vi "MOPX2 Engine.vi"(8 "Operation Selection":T1, 9 "Main Parent  MO4J":u16[][](array[numeric]), 10 "Secondary Parent Schedule":u16[](array[numeric]), 11 "Main Parent Schedule":u16[](array[numeric])) -> (3 "Child Schedule":u16[](array[numeric]))   [LabVIEW 2013, in "GA.lvclass"]
uses:
  GA.lvclass
  Controls/MPOX2 Operation Selection Rule.ctl
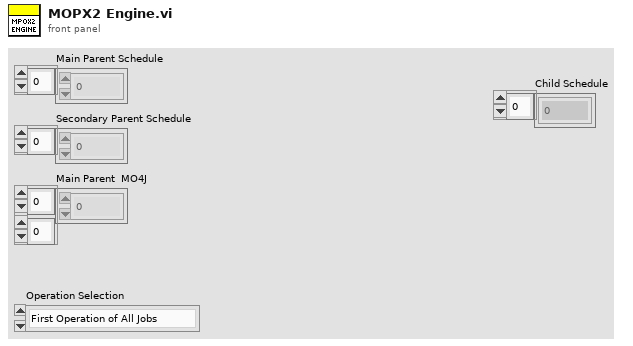
[diagram p1: front panel]
types:
  T1 = typedef "GA.lvclass/MPOX2 Operation Selection Rule.ctl" = enum16{"First Operation of All Jobs", "Random"}
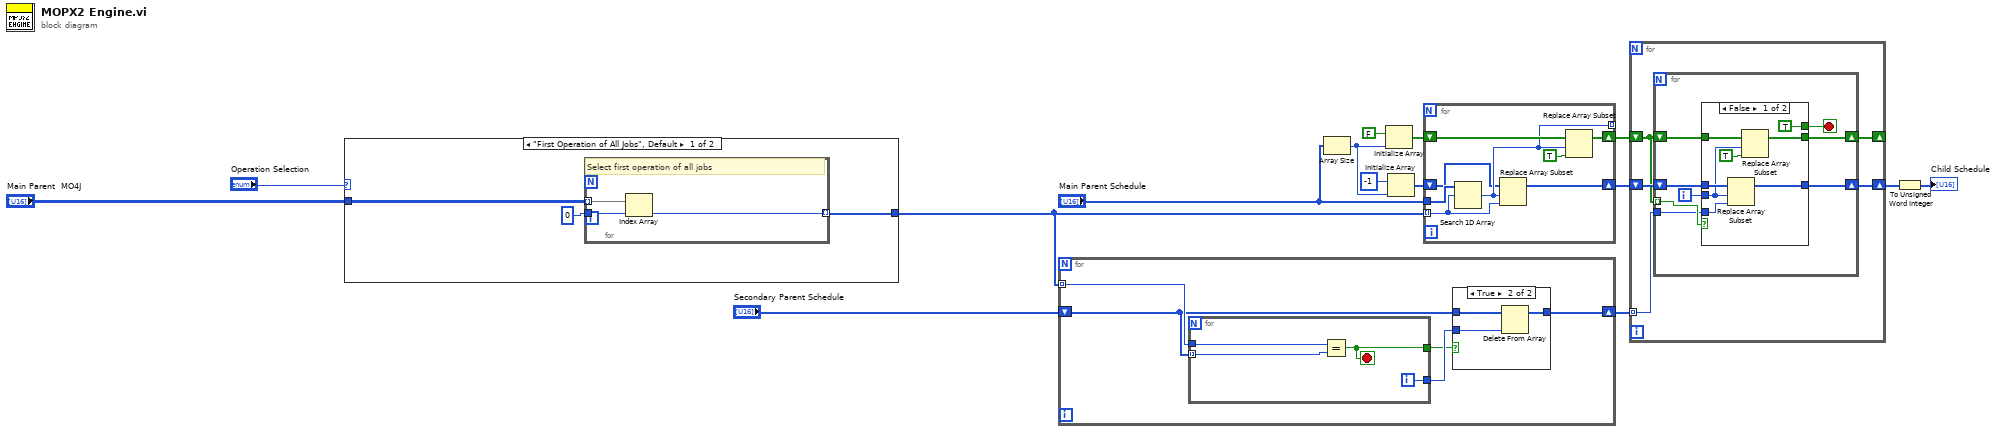
[diagram p0: block diagram]
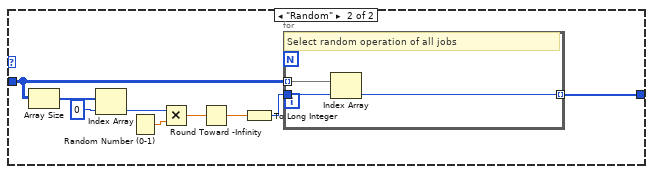
[diagram p2: hidden frame]
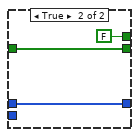
[diagram p3: hidden frame]
diagram:
  n1 = case shown="\"First Operation of All Jobs\", Default" "Operation Selection" {
    tunnel: "Main Parent  MO4J" -> [w18 w30]
    tunnel: [w17 w22] -> w2
    frame "First Operation of All Jobs", Default {
      n2 = for {
        tunnel: w18 -> [w21] mode=indexing
        tunnel: [w20] -> w17 mode=indexing
        tunnel: 0 ("index") -> [w19]
        # "Select first operation of all jobs"
        n3 = Index Array(array=w21, index=w19) -> (element=w20:u16)
      }
    }
    frame "Random" {
      n4 = Array Size(array=w30) -> (size(s)=w29:i32[])
      n5 = Index Array(array=w29, index=0) -> (element=w27:i32)
      n6 = Random Number (0-1)() -> (number: 0 to 1=w26:dbl)
      n7 = Multiply(x=w27, y=w26) -> (x*y=w25:dbl)
      n8 = Round Toward -Infinity(1:w25) -> (0:w24:dbl)
      n9 = To Long Integer(number=w24) -> (32bit integer=w23:i32)
      n10 = for {
        tunnel: w30 -> [w33] mode=indexing
        tunnel: [w32] -> w22 mode=indexing
        tunnel: w23 -> [w31]
        # "Select random operation of all jobs"
        n11 = Index Array(array=w33, index=w31) -> (element=w32:u16)
      }
    }
  }
  n12 = for {
    tunnel: w2 -> [w38] mode=indexing
    shift-right: [w35] -> w5
    shift-left: "Secondary Parent Schedule" -> [w37]
    n13 = for {
      tunnel: w37 -> [w45] mode=indexing
      tunnel: w38 -> [w46]
      tunnel: [w44] -> w36
      tunnel: [w43] -> w34
      i -> [w44]
      stop <- w43 stop-if-true
      n14 = Equal?(x=w46, y=w45) -> (x = y?=w43:bool)
    }
    n15 = case shown="True" w34 {
      tunnel: w37 -> [w39 w42]
      tunnel: w36 -> [_ w41]
      tunnel: [w39 w40] -> w35
      frame False {
      }
      frame True {
        n16 = Delete From Array(array=w42, index=w41) -> (array with subset deleted=w40:u16[])  [unwired: 1 in, 1 out]
      }
    }
  }
  n17 = Array Size(array="Main Parent Schedule") -> (size(s)=w11:i32)
  n18 = Initialize Array(FALSE, w11) -> (w13:bool[])
  n19 = Initialize Array(-1, w11) -> (w9:i32[])
  n20 = for {
    tunnel: "Main Parent Schedule" -> [w54]
    tunnel: w2 -> [w50] mode=indexing
    tunnel: [w51] -> _ mode=indexing
    shift-right: [w47] -> w7
    shift-left: w13 -> [w53]
    shift-right: [w48] -> w6
    shift-left: w9 -> [w49]
    n21 = Search 1D Array(1D array=w54, element=w50) -> (index of element=w51:i32)  [unwired: 1 in]
    n22 = Replace Array Subset(array=w49, new element=w50, index=w51) -> (w48:i32[])
    n23 = Replace Array Subset(array=w53, new element=TRUE ("new element/subarray"), index=w51) -> (w47:bool[])
  }
  n24 = for {
    tunnel: w5 -> [w59] mode=indexing
    shift-right: [w57] -> w4
    shift-left: w6 -> [w58]
    shift-right: [w55] -> _
    shift-left: w7 -> [w56]
    n25 = for {
      tunnel: w56 -> [w67] mode=indexing
      tunnel: w59 -> [w64]
      shift-right: [w65] -> w57
      shift-left: w58 -> [w66]
      shift-right: [w61] -> w55
      shift-left: w56 -> [w62]
      i -> [w63]
      stop <- w60 stop-if-true
      n26 = case shown="False" w67 {
        tunnel: w66 -> [w75 w78]
        tunnel: [w73 w78] -> w65
        tunnel: w64 -> [w74 _]
        tunnel: w63 -> [w71 _]
        tunnel: w62 -> [w72 w77]
        tunnel: [w69 w77] -> w61
        tunnel: [TRUE FALSE] -> w60
        frame False {
          n27 = Replace Array Subset(array=w75, new element=w74, index=w71) -> (w73:i32[])
          n28 = Replace Array Subset(array=w72, new element=TRUE ("new element/subarray"), index=w71) -> (w69:bool[])
        }
        frame True {
        }
      }
    }
  }
  n29 = To Unsigned Word Integer(number=w4) -> (unsigned 16bit integer=→"Child Schedule":u16[])
